vi "AutoListProcessor.vi"(11 "AutoList":T1[](array[typedef])) -> ()   [LabVIEW 2023]
uses:
  Elevator/ElevatorSetpointEnum.ctl
  ClusterEnumTypedef.ctl
  ClusterTypedef.ctl
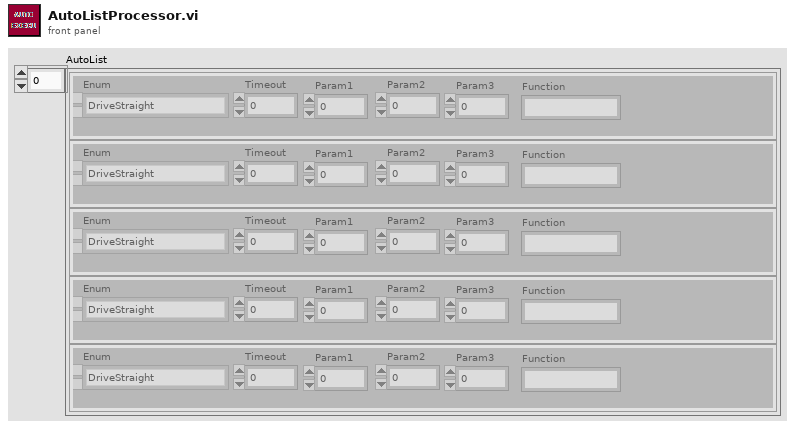
[diagram p1: front panel]
types:
  T1 = typedef "ClusterTypedef.ctl" = cluster{"Enum":T2, "Timeout":dbl, "Param1":dbl, "Param2":dbl, "Param3":dbl, "Function":string}
  T2 = typedef "ClusterEnumTypedef.ctl" = enum16{"DriveStraight", "DriveTurn", "FollowAbsoluteTrajectory", "FollowRelativeTrajectory", "AutoWait", "ElevToRest", "ElevToSource", "ElevToL1", "ElevToL2", "ElevToL3", "ElevToL4", "ElevToAlgae1", "ElevToAlgae2", "ElevCancel", "IntakeCoral", "IntakeAlgae", "IntakeDepositCoral", "IntakeDepositAlgae", "IntakeCancel", "ElevRestWait", "ElevSourceWait", "ElevL1Wait", "ElevL2Wait", "ElevAlgae1Wait", "ElevL3Wait", "ElevAlgae2Wait", "ElevL4Wait"}
  T3 = typedef "ElevatorSetpointEnum.ctl" = enum16{"Rest", "Source", "L1", "L2", "Algae1", "L3", "Algae2", "L4"}
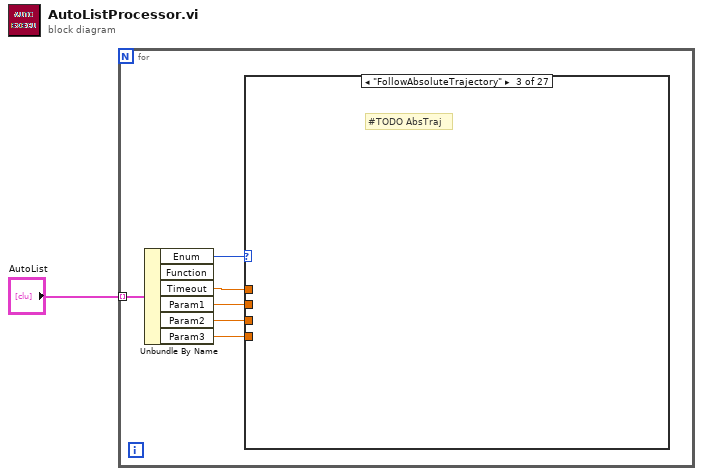
[diagram p0: block diagram]
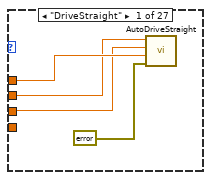
[diagram p2: hidden frame]
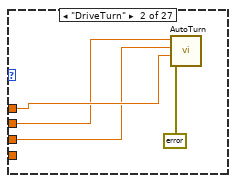
[diagram p3: hidden frame]
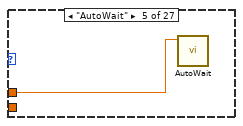
[diagram p5: hidden frame]
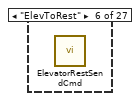
[diagram p6: hidden frame]
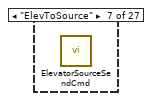
[diagram p7: hidden frame]
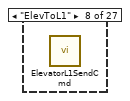
[diagram p8: hidden frame]
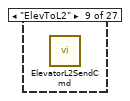
[diagram p9: hidden frame]
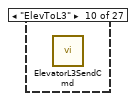
[diagram p10: hidden frame]
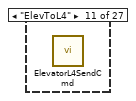
[diagram p11: hidden frame]
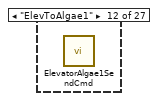
[diagram p12: hidden frame]
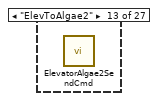
[diagram p13: hidden frame]
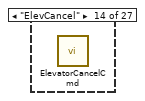
[diagram p14: hidden frame]
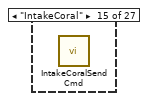
[diagram p15: hidden frame]
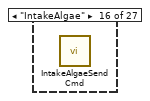
[diagram p16: hidden frame]
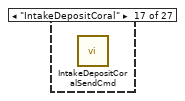
[diagram p17: hidden frame]
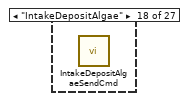
[diagram p18: hidden frame]
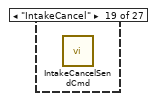
[diagram p19: hidden frame]
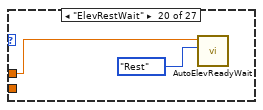
[diagram p20: hidden frame]
diagram:
  n1 = for {
    tunnel: "AutoList" -> [w7] mode=indexing
    n2 = Unbundle By Name(w7) -> ("Enum"=w6:T2, "Timeout"=w5:dbl, "Param1"=w4:dbl, "Param2"=w2:dbl, "Param3"=w3:dbl)  [unwired: 1 out]
    n3 = case shown="\"FollowAbsoluteTrajectory\"" w6 {
      tunnel: w5 -> [w11 w15 _ _ w16 _ _ _ _ _ _ _ _ _ _ _ _ _ _ w17 w19 w21 w23 w25 w27 w29 w31]
      tunnel: w4 -> [w10 w14 _ _ _ _ _ _ _ _ _ _ _ _ _ _ _ _ _ _ _ _ _ _ _ _ _]
      tunnel: w3 -> [_ _ _ _ _ _ _ _ _ _ _ _ _ _ _ _ _ _ _ _ _ _ _ _ _ _ _]
      tunnel: w2 -> [w9 w13 _ _ _ _ _ _ _ _ _ _ _ _ _ _ _ _ _ _ _ _ _ _ _ _ _]
      frame "DriveStraight" {
        n4 = call "AutoDriveStraight.vi"("error in (no error)"=errorcluster {"status"=FALSE, "code"=0, "source"=""}, "TimeOut (s)"=w11, "MaxSpeed (ft/s)"=w9, "Dist (ft)"=w10) -> ()  [unwired: 7 in, 1 out]
      }
      frame "DriveTurn" {
        n5 = call "AutoTurn.vi"("error in (no error)"=errorcluster {"status"=FALSE, "code"=0, "source"=""}, "TimeOut (s)"=w15, "MaxSpeed (ft/s)"=w13, "degrees"=w14) -> ()  [unwired: 7 in, 1 out]
      }
      frame "FollowAbsoluteTrajectory" {
        # "#TODO AbsTraj"
      }
      frame "FollowRelativeTrajectory" {
        # "#TODO Follow Rel traj"
      }
      frame "AutoWait" {
        n6 = call "AutoWait.vi"("TimeOut (s)"=w16) -> ()  [unwired: 10 in, 1 out]
      }
      frame "ElevToRest" {
        n7 = call "ElevatorRestSendCmd.vi"() -> ()  [unwired: 11 in, 1 out]
      }
      frame "ElevToSource" {
        n8 = call "ElevatorSourceSendCmd.vi"() -> ()  [unwired: 11 in, 1 out]
      }
      frame "ElevToL1" {
        n9 = call "ElevatorL1SendCmd.vi"() -> ()  [unwired: 11 in, 1 out]
      }
      frame "ElevToL2" {
        n10 = call "ElevatorL2SendCmd.vi"() -> ()  [unwired: 11 in, 1 out]
      }
      frame "ElevToL3" {
        n11 = call "ElevatorL3SendCmd.vi"() -> ()  [unwired: 11 in, 1 out]
      }
      frame "ElevToL4" {
        n12 = call "ElevatorL4SendCmd.vi"() -> ()  [unwired: 11 in, 1 out]
      }
      frame "ElevToAlgae1" {
        n13 = call "ElevatorAlgae1SendCmd.vi"() -> ()  [unwired: 11 in, 1 out]
      }
      frame "ElevToAlgae2" {
        n14 = call "ElevatorAlgae2SendCmd.vi"() -> ()  [unwired: 11 in, 1 out]
      }
      frame "ElevCancel" {
        n15 = call "ElevatorCancelCmd.vi"() -> ()  [unwired: 11 in, 1 out]
      }
      frame "IntakeCoral" {
        n16 = call "IntakeCoralSendCmd.vi"() -> ()  [unwired: 11 in, 1 out]
      }
      frame "IntakeAlgae" {
        n17 = call "IntakeAlgaeSendCmd.vi"() -> ()  [unwired: 11 in, 1 out]
      }
      frame "IntakeDepositCoral" {
        n18 = call "IntakeDepositCoralSendCmd.vi"() -> ()  [unwired: 11 in, 1 out]
      }
      frame "IntakeDepositAlgae" {
        n19 = call "IntakeDepositAlgaeSendCmd.vi"() -> ()  [unwired: 11 in, 1 out]
      }
      frame "IntakeCancel" {
        n20 = call "IntakeCancelSendCmd.vi"() -> ()  [unwired: 11 in, 1 out]
      }
      frame "ElevRestWait" {
        n21 = call "AutoElevReadyWait.vi"("ElevatorSetpoints"=ElevatorSetpointEnum."Rest", "TimeOut (s)"=w17) -> ()  [unwired: 9 in, 1 out]
      }
      frame "ElevSourceWait" {
        n22 = call "AutoElevReadyWait.vi"("ElevatorSetpoints"=ElevatorSetpointEnum."Source", "TimeOut (s)"=w19) -> ()  [unwired: 9 in, 1 out]
      }
      frame "ElevL1Wait" {
        n23 = call "AutoElevReadyWait.vi"("ElevatorSetpoints"=ElevatorSetpointEnum."L1", "TimeOut (s)"=w21) -> ()  [unwired: 9 in, 1 out]
      }
      frame "ElevL2Wait" {
        n24 = call "AutoElevReadyWait.vi"("ElevatorSetpoints"=ElevatorSetpointEnum."L2", "TimeOut (s)"=w23) -> ()  [unwired: 9 in, 1 out]
      }
      frame "ElevAlgae1Wait" {
        n25 = call "AutoElevReadyWait.vi"("ElevatorSetpoints"=ElevatorSetpointEnum."Algae1", "TimeOut (s)"=w25) -> ()  [unwired: 9 in, 1 out]
      }
      frame "ElevL3Wait" {
        n26 = call "AutoElevReadyWait.vi"("ElevatorSetpoints"=ElevatorSetpointEnum."L3", "TimeOut (s)"=w27) -> ()  [unwired: 9 in, 1 out]
      }
      frame "ElevAlgae2Wait" {
        n27 = call "AutoElevReadyWait.vi"("ElevatorSetpoints"=ElevatorSetpointEnum."Algae2", "TimeOut (s)"=w29) -> ()  [unwired: 9 in, 1 out]
      }
      frame "ElevL4Wait" {
        n28 = call "AutoElevReadyWait.vi"("ElevatorSetpoints"=ElevatorSetpointEnum."L4", "TimeOut (s)"=w31) -> ()  [unwired: 9 in, 1 out]
      }
    }
  }
